vi "APS Release simultaneous move.vi"(8 "error in (no error)":errorcluster caption="错误输入（无错误）", 11 "Axis_ID":i32) -> (0 "error out":errorcluster caption="错误输出", 3 "function return":i32)   [LabVIEW 2011, in "APS168.lvlib"]
doc: "I32 FNTYPE APS_release_simultaneous_move ( I32 Axis_ID );"
uses:
  APS168.lvlib
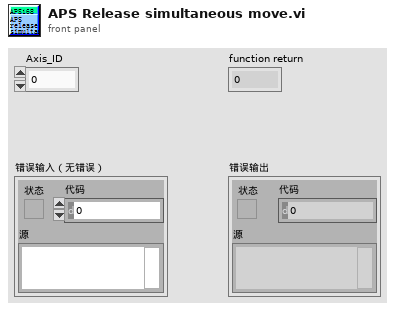
[diagram p1: front panel]
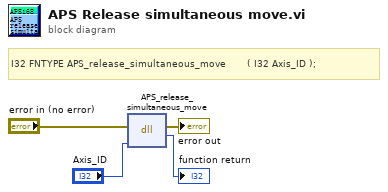
[diagram p0: block diagram]
diagram:
  # "I32 FNTYPE APS_release_simultaneous_move       ( I32 Axis_ID );"
  n1 = dll-call lib="PTH1Labs E软件ADLINK 204CAPS_1_7_1_LIB line 连续运动204APS168.*" fn="APS_release_simultaneous_move"(error in="error in (no error)", "Axis_ID"="Axis_ID") -> (error out=→"error out":errorcluster, →"function return":i32)  [unwired: 3 in, 1 out]
